vi "RegisterMap to Table Entries.vi"(5 "get unmapped?":bool, 7 "get mapped?":bool, 8 "error in (no error)":errorcluster, 9 "Indicators RegisterMap":T1[](array[typedef]) {"Address" format="%.0x"}, 10 "input type":string, 11 "Item Ref in":T6 format="%.0x") -> (0 "error out":errorcluster, 2 "Table Entries":T7[](array[typedef]) {"FPGA CD Ref" format="%.0x"; "reserver" format="%.0x"})   [LabVIEW 2016, in "FPGA Resource Manager System Definition.lvlib"]
uses:
  FPGA Resource Manager System Definition.lvlib
  resource info.ctl
  <vilib>/NI Veristand/Custom Device API/Custom Device Item Ref.ctl
  <vilib>/rvi/Bitfile/nirviControlStructure.ctl
  <vilib>/rvi/Bitfile/nirviTypdefDescription.ctl
  <vilib>/rvi/Bitfile/nirviMechanicalAction.ctl
  <vilib>/rvi/Bitfile/nirviSubControlStructure.ctl
  <vilib>/rvi/Bitfile/nirviClusterElementControl.ctl
  FPGA-Addon/Source/System Explorer/FPGA Addon System Explorer.lvlib
  <vilib>/NI VeriStand/Custom Device API/Custom Device API.lvlib
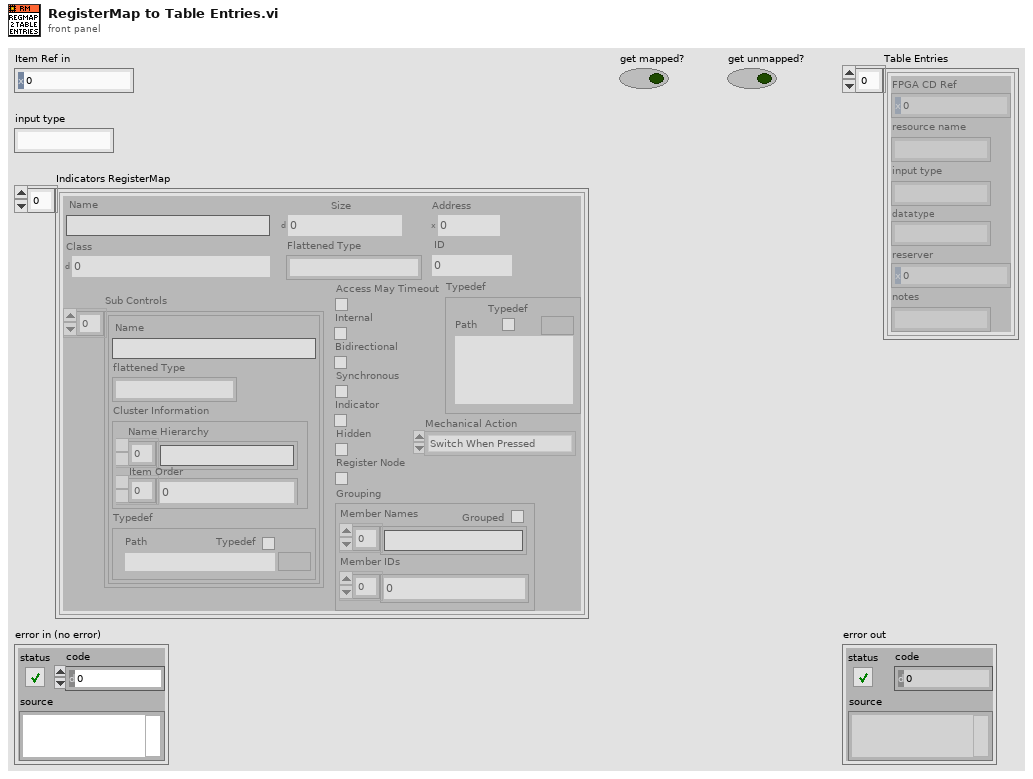
[diagram p1: front panel]
types:
  T1 = typedef "nirviControlStructure.ctl" = cluster{"Name":string, "Hidden":bool, "Indicator":bool, "Flattened Type":string, "Grouping":cluster{"Grouped":bool, "Member Names":string[], "Member IDs":u32[]}, "Address":u32, "Size":u32, "Class":u32, "Internal":bool, "Typedef":T2, "ID":u32, "Bidirectional":bool, "Synchronous":bool, "Mechanical Action":T3, "Sub Controls":T4[], "Access May Timeout":bool, "Register Node":bool}
  T2 = typedef "nirviTypdefDescription.ctl" = cluster{"Typedef":bool, "Path":path}
  T3 = typedef "nirviMechanicalAction.ctl" = enum8{"Switch When Pressed", "Switch When Released", "Switch Until Released", "Latch When Pressed", "Latch When Released", "Latch Until Released"}
  T4 = typedef "nirviSubControlStructure.ctl" = cluster{"Name":string, "flattened Type":string, "Cluster Information":T5, "Typedef":T2}
  T5 = typedef "nirviClusterElementControl.ctl" = cluster{"Name Hierarchy":string[], "Item Order":u32[]}
  T6 = typedef "Custom Device API.lvlib/Custom Device Item Ref.ctl" = u64
  T7 = typedef "FPGA Resource Manager System Definition.lvlib/resource info.ctl" = cluster{"FPGA CD Ref":T6, "resource name":string, "input type":string, "datatype":string, "reserver":T6, "notes":string}
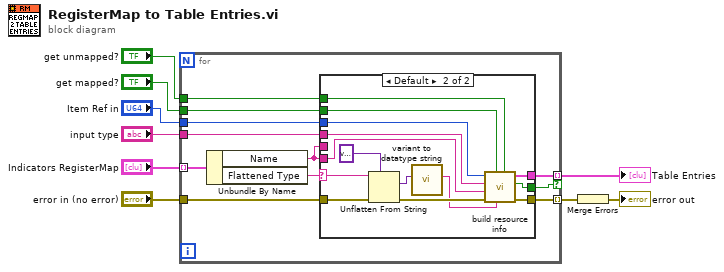
[diagram p0: block diagram]
diagram:
  n1 = for {
    tunnel: "Indicators RegisterMap" -> [w20] mode=indexing
    tunnel: "Item Ref in" -> [w19]
    tunnel: "get mapped?" -> [w18]
    tunnel: "get unmapped?" -> [w17]
    tunnel: [w15] -> w8 mode=indexing if=w12
    tunnel: "input type" -> [w14]
    tunnel: "error in (no error)" -> [w11]
    tunnel: [w13] -> w2 mode=indexing
    n2 = Unbundle By Name(w20) -> ("Name"=w10:string, "Flattened Type"=w16:string)
    n3 = case shown="Default" w16 {
      selector: w16 -> [_ w31]
      tunnel: w19 -> [_ w35]
      tunnel: w18 -> [_ w34]
      tunnel: w17 -> [_ w33]
      tunnel: w10 -> [_ w32]
      tunnel: [_ w30] -> w15
      tunnel: w14 -> [_ w29]
      tunnel: [w21 w28] -> w13
      tunnel: [_ w27] -> w12
      tunnel: w11 -> [w21 w26]
      tunnel: w10 -> [_ _]
      frame "" {
      }
      frame Default {
        n4 = Unflatten From String(type=variant, binary string=w31, error in (no error)=w26) -> (value=w24:variant, error out=w23:errorcluster)  [unwired: 2 in, 1 out]
        n5 = call "variant to datatype string.vi"("Variant"=w24) -> ("datatype string"=w22:string)  [unwired: 9 in, 1 out]
        n6 = call "build resource info.vi"("get unmapped?"=w33, "datatype"=w22, "get mapped?"=w34, "error in (no error)"=w23, "name in bitfile"=w32, "input type"=w29, "FPGA CD Ref"=w35) -> ("error out"=w28:errorcluster, "include?"=w27:bool, "visualizer entry"=w30:T7)  [unwired: 2 in]
      }
    }
  }
  "Table Entries" <- w8
  n7 = Merge Errors(w2) -> (→"error out":errorcluster)
